vi "Runge Kutta Check Prep.vi"(2 "F(X,t) coded":i32[](array[numeric]), 3 "time":string, 4 "X coded":i32[](array[numeric])) -> (0 "number of X variables":i32, 1 "variables correct?":bool)   [LabVIEW 2020, in "NI_Gmath.lvlib"]
uses:
  <vilib>/gmath/NI_Gmath.lvlib
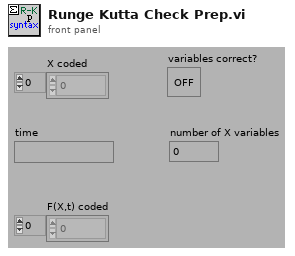
[diagram p1: front panel]
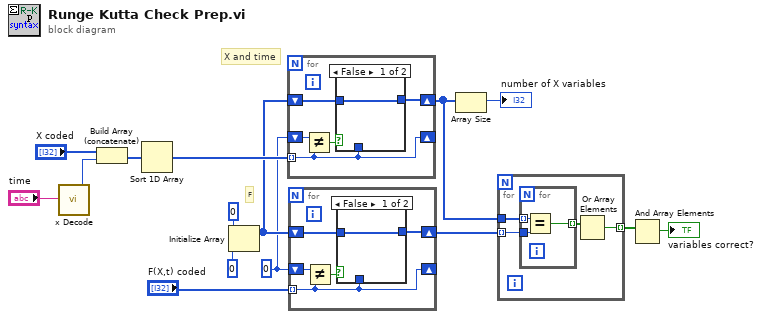
[diagram p0: block diagram]
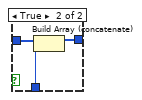
[diagram p2: hidden frame]
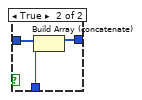
[diagram p3: hidden frame]
diagram:
  w3 = 0
  # "X and time"
  # "F"
  n1 = call <vilib>:"x Decode.vi"("x string"="time") -> ("number"=w6:i32)  [unwired: 1 in, 1 out]
  n2 = Build Array (concatenate)("X coded", w6) -> (w8:i32[])
  n3 = Sort 1D Array(array=w8) -> (sorted array=w9:i32[])
  n4 = Initialize Array(0, 0) -> (w7:i32[])
  n5 = for {
    shift-right: [w17] -> w12
    shift-left: w7 -> [w18]
    shift-right: [w16] -> _
    shift-left: w3 -> [w20]
    tunnel: w9 -> [w16] mode=indexing
    n6 = Not Equal?(x=w20, y=w16) -> (x != y?=w19:bool)
    n7 = case shown="False" w19 {
      tunnel: w18 -> [w21 w24]
      tunnel: [w21 w23] -> w17
      tunnel: w16 -> [_ w22]
      frame False {
      }
      frame True {
        n8 = Build Array (concatenate)(w24, w22) -> (w23:i32[])
      }
    }
  }
  n9 = for {
    shift-right: [w26] -> w11
    shift-left: w7 -> [w27]
    shift-right: [w25] -> _
    shift-left: w3 -> [w29]
    tunnel: "F(X,t) coded" -> [w25] mode=indexing
    n10 = Not Equal?(x=w29, y=w25) -> (x != y?=w28:bool)
    n11 = case shown="False" w28 {
      tunnel: w27 -> [w30 w33]
      tunnel: [w30 w32] -> w26
      tunnel: w25 -> [_ w31]
      frame False {
      }
      frame True {
        n12 = Build Array (concatenate)(w33, w31) -> (w32:i32[])
      }
    }
  }
  n13 = Array Size(array=w12) -> (size(s)=→"number of X variables":i32)
  n14 = for {
    tunnel: w11 -> [w37] mode=indexing
    tunnel: w12 -> [w36]
    tunnel: [w34] -> w13 mode=indexing
    n15 = for {
      tunnel: w37 -> [w40]
      tunnel: w36 -> [w39] mode=indexing
      tunnel: [w38] -> w35 mode=indexing
      n16 = Equal?(x=w39, y=w40) -> (x = y?=w38:bool)
    }
    n17 = Or Array Elements(Boolean array=w35) -> (logical OR=w34:bool)
  }
  n18 = And Array Elements(Boolean array=w13) -> (logical AND=→"variables correct?":bool)
